vi "Lookup Node (Target Group).vi"(8 "error in (no error)":errorcluster, 10 "Target Name":string, 11 "Cluster in":refnum<class "Cluster Config.lvclass">) -> (0 "error out":errorcluster, 2 "Nodes":refnum<class "Node Config.lvclass">[](array[class]), 3 "Cluster out":refnum<class "Cluster Config.lvclass">)   [LabVIEW 2020, in "VolatusConfig.lvlib" / "Cluster Config.lvclass"]
uses:
  Cluster Config.lvclass
  C:/dev/lv20CE/relink/lv-volatus/VolatusConfig/VolatusConfigElement/VolatusConfigElement.lvclass
  Meta Type.ctl
  VolatusConfigElement/VolatusConfigElement.lvclass/VolatusConfigElement.ctl
  VolatusConfigElement/Element.vi
  lv-cdm/CDM-Config/Config Lookup/Match Meta.vi
  lv-cdm/CDM-Config/Config Element/Owner.vi
  lv-cdm/CDM-Config/Config Manager/Lookup Descendant.vi
  lv-cdm/CDM-Config/Config Element/Name.vi
  lv-cdm/CDM-Config/Config Filter/Config Lookup.lvclass
  Cluster Config.lvclass/Cluster Config.ctl
  VolatusConfigElement/VolatusConfigElement.lvclass
  VolatusConfig.lvlib
  Node/Node Config.lvclass
  C:/dev/lv20CE/relink/lv-volatus/VolatusConfig/Cluster/Cluster Config.lvclass
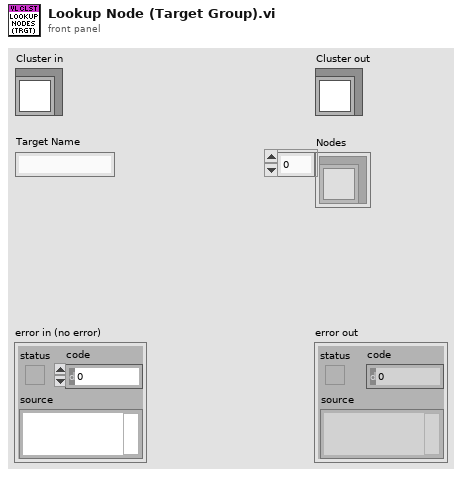
[diagram p1: front panel]
types:
  T1 = typedef "VolatusConfig.lvlib/Meta Type.ctl" = enum16{"UNKNOWN", "VL_System", "VL_Cluster", "VL_Node", "VL_Task", "VL_Group", "VL_Channel", "VL_Task_List", "VL_Scaling", "VL_Sensor", "VL_Sensor_List", "VL_Scale"}
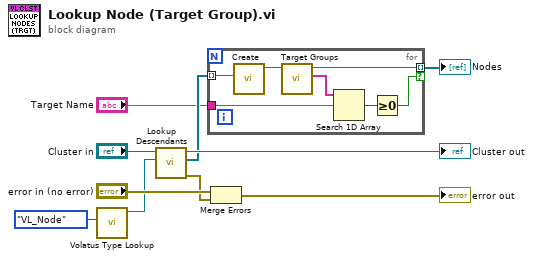
[diagram p0: block diagram]
diagram:
  n1 = call "Volatus Type Lookup.vi"("Meta Type"=Meta_Type."VL_Node") -> ("Config Lookup out"=w5:refnum<class "Config Lookup.lvclass">)  [unwired: 9 in, 1 out]
  n2 = call "Lookup Descendants.vi"("Lookup"=w5, "VolatusConfigElement in"="Cluster in") -> ("error out"=w1:errorcluster, "Descendants"=w4:refnum<class "Config Element.lvclass">[], "VolatusConfigElement out"=→"Cluster out":refnum<class "Cluster Config.lvclass">)  [unwired: 7 in]
  n3 = for {
    tunnel: w4 -> [w17] mode=indexing
    tunnel: "Target Name" -> [w14]
    tunnel: [w13] -> w2 mode=indexing if=w11
    n4 = call "Create.vi"("Element"=w17) -> ("Node out"=w16:refnum<class "Node Config.lvclass">)  [unwired: 9 in, 1 out]
    n5 = call "Target Groups.vi"("Node in"=w16) -> ("Target Groups"=w15:string[], "Node out"=w13:refnum<class "Node Config.lvclass">)  [unwired: 8 in, 1 out]
    n6 = Search 1D Array(1D array=w15, element=w14) -> (index of element=w12:i32)  [unwired: 1 in]
    n7 = Greater Or Equal To 0?(x=w12) -> (x >= 0?=w11:bool)
  }
  "Nodes" <- w2
  n8 = Merge Errors("error in (no error)", w1) -> (→"error out":errorcluster)
